vi "Create Linear Waveform.vi"(8 "dt":dbl=10.0 max=1.0 step=0.01, 9 "Period":dbl=10.0 format="%.2g", 10 "V Start":dbl, 11 "V End":dbl) -> (3 "signal out":waveform(dbl))   [LabVIEW 2018]
uses:
  <vilib>/measure/NI_MAPro.lvlib
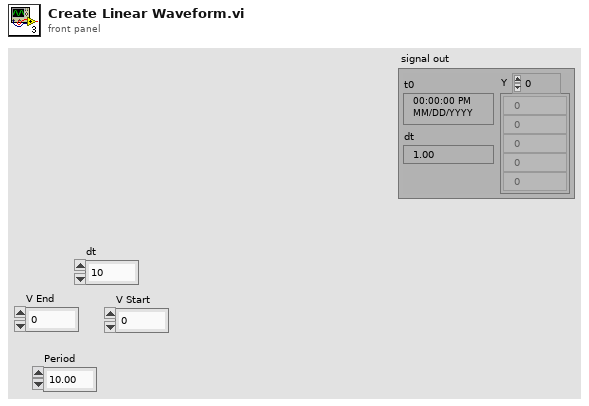
[diagram p1: front panel]
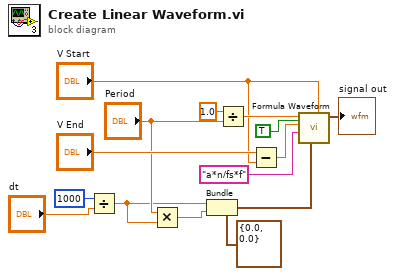
[diagram p0: block diagram]
diagram:
  n1 = Divide(x=u32 1000 ("y"), y="dt") -> (x/y=w3:dbl)
  n2 = Multiply(x="Period", y=w3) -> (x*y=w10:dbl)
  n3 = Bundle(cluster=cluster{dbl, dbl} {0.0, 0.0} ("input cluster"), w3, w10) -> (w7:cluster{dbl, dbl})
  n4 = Divide(x=1.0, y="Period") -> (x/y=w8:dbl)
  n5 = Subtract(x="V End", y="V Start") -> (x-y=w5:dbl)
  n6 = call <vilib>:"Formula Waveform.vi"("offset"="V Start", "sampling info"=w7, "reset signal"=TRUE, "formula"="a*n/fs*f", "amplitude"=w5, "frequency"=w8) -> ("signal out"=→"signal out":waveform(dbl))  [unwired: 4 in, 1 out]
